vi "Get niRfsgBT Handle.vi"(8 "error in (no error)":errorcluster, 11 "niDTS BT INSTR RX in":refnum<class "niDTS BT INSTR RX.lvclass">) -> (0 "error out":errorcluster, 2 "InstDriver Handle in":T1, 3 "niDTS BT INSTR RX out":refnum<class "niDTS BT INSTR RX.lvclass">)   [LabVIEW 2015, in "niDTS BT.lvlib" / "niDTS BT INSTR RX.lvclass"]
uses:
  niDTS BT INSTR RX.lvclass
  RiviInstDriver/niRfsgBT/Includes/niRfsgBt INC Handle.ctl
  RiviInstDriver/niRfsgBT/Objects/niRfsgBt.lvclass
  niDTS BT INSTR RX.lvclass/niDTS BT INSTR RX.ctl
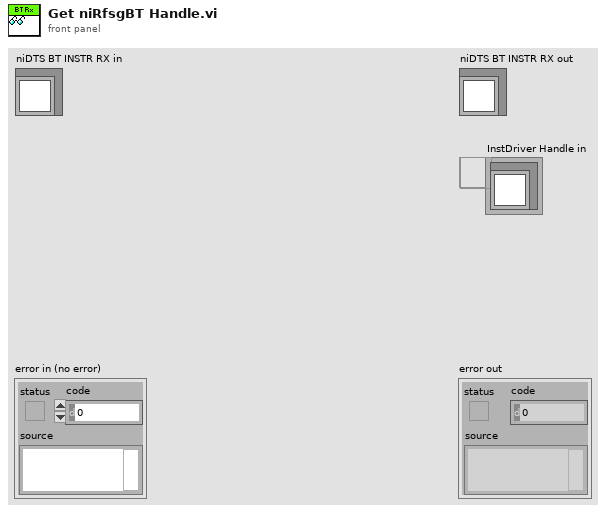
[diagram p1: front panel]
types:
  T1 = typedef "niRfsgBT.lvclass/niRfsgBT INC Handle.ctl" = refnum<data-value>
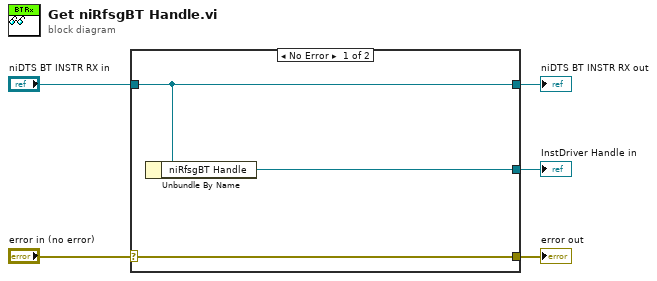
[diagram p0: block diagram]
diagram:
  n1 = case shown="No Error" "error in (no error)" {
    selector: "error in (no error)" -> [w8 w9]
    tunnel: [w8 w9] -> w4
    tunnel: [w7 w10] -> w2
    tunnel: "niDTS BT INSTR RX in" -> [w7 w10]
    tunnel: [w6 _] -> w1
    frame No Error {
      n2 = Unbundle By Name(w7) -> ("niRfsgBT Handle"=w6:T1)
    }
    frame Error {
    }
  }
  "error out" <- w4
  "niDTS BT INSTR RX out" <- w2
  "InstDriver Handle in" <- w1
